vi "Get Types for Worker.vi"(11 "Worker VI In":refnum<vi>) -> (1 "Types":T2[](array[typedef]), 2 "Special Terminals":T1={"Action"=-1, "Init"=-1, "Tag"=-1, "State in"=-1, "State out"=-1, "Error"=-1}, 3 "Worker VI":refnum<vi>)   [LabVIEW 2020, in "FlexBlocks.lvlib"]
uses:
  FlexBlocks.lvlib
  Special Terminal Indices.ctl
  Worker Action.ctl
  <vilib>/Utility/Data Type/NI_Data Type.lvlib
  Terminal Direction.ctl
  Value Mode.ctl
  Special Terminal.ctl
  Type Descriptor.ctl
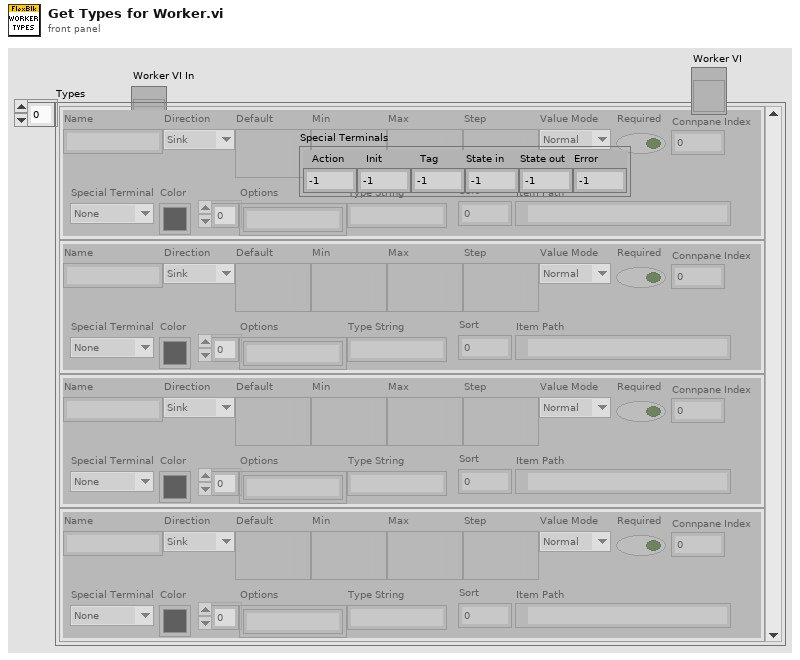
[diagram p1: front panel]
types:
  T1 = typedef "FlexBlocks.lvlib/Special Terminal Indices.ctl" = cluster{"Action":i32, "Init":i32, "Tag":i32, "State in":i32, "State out":i32, "Error":i32}
  T2 = typedef "FlexBlocks.lvlib/Type Descriptor.ctl" = cluster{"Name":string, "Direction":T3, "Default":variant, "Min":variant, "Max":variant, "Step":variant, "Value Mode":T4, "Required":bool, "Connpane Index":i32, "Special Terminal":T5, "Color":u32, "Options":string[], "Type String":string, "Sort":i32, "Item Path":path}
  T3 = typedef "FlexBlocks.lvlib/Terminal Direction.ctl" = enum16{"Sink", "Source"}
  T4 = typedef "FlexBlocks.lvlib/Value Mode.ctl" = enum16{"Normal", "Range", "Select"}
  T5 = typedef "FlexBlocks.lvlib/Special Terminal.ctl" = enum16{"None", "Action", "Init", "Tag", "State in", "State out", "Error"}
  T6 = typedef "FlexBlocks.lvlib/Worker Action.ctl" = enum16{"Start", "Work", "Stop"}
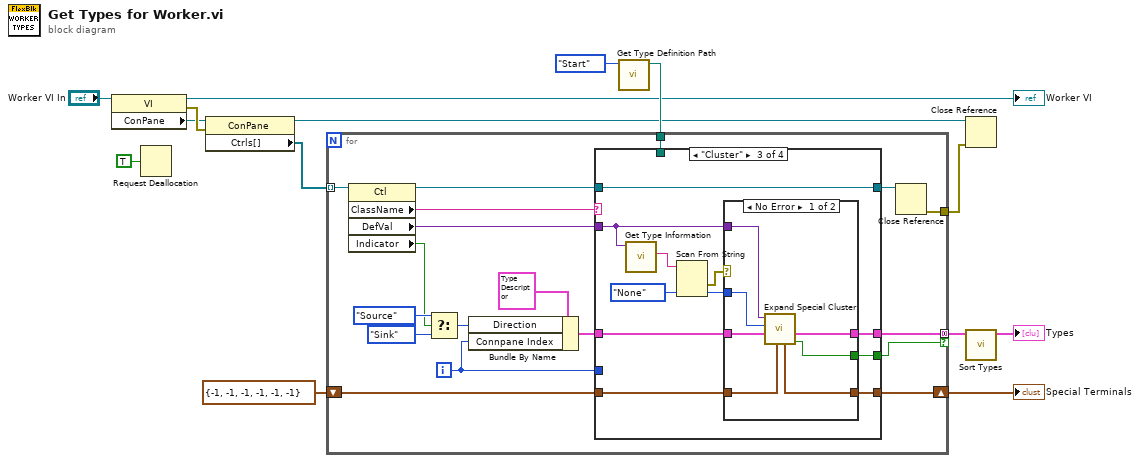
[diagram p0: block diagram]
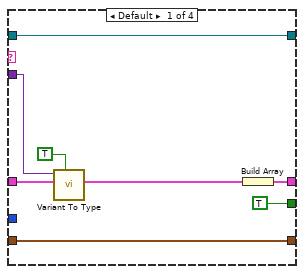
[diagram p2: hidden frame]
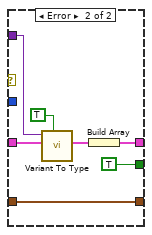
[diagram p4: hidden frame]
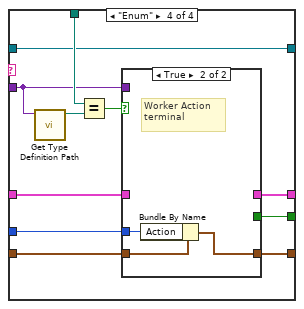
[diagram p5: hidden frame]
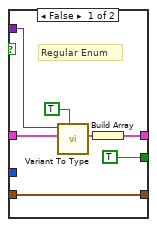
[diagram p6: hidden frame]
diagram:
  n1 = property class="VI"(reference="Worker VI In") -> (reference out=→"Worker VI":refnum<vi>, error out=w14:errorcluster, "ConPane"=w13:refnum<vi>)  [unwired: 1 in]
  n2 = Request Deallocation(TRUE ("flag")) -> ()
  n3 = property class="ConPane"(reference=w13, error in=w14) -> (reference out=w6:refnum<vi>, "Ctrls[]"=w10:refnum<vi>[])  [unwired: 1 out]
  n4 = call <vilib>:"Get Type Definition Path.vi"("variant"=Worker_Action."Start" ("Action")) -> ("type definition path"=w7:path)  [unwired: 9 in, 1 out]
  n5 = for {
    tunnel: w10 -> [w32] mode=indexing
    shift-right: [w18] -> w3
    shift-left: T1 {"Action"=-1, "Init"=-1, "Tag"=-1, "State in"=-1, "State out"=-1, "Error"=-1} ("Special Term Indices") -> [w19]
    tunnel: w7 -> [w17]
    tunnel: [w21] -> w4 mode=concatenating if=w20
    tunnel: [w15] -> w5
    i -> [w23]
    n6 = property class="Ctl"(reference=w32) -> (reference out=w30:refnum<vi>, "ClassName"=w31:string, "DefVal"=w29:variant, "Indicator"=w26:bool)  [unwired: 1 in, 1 out]
    n7 = Select(t=Terminal_Direction."Source" ("Direction"), s=w26, f=Terminal_Direction."Sink" ("Direction")) -> (s? t:f=w24:T3)
    n8 = Bundle By Name(cluster=T2 {"Name"="", "Direction"=enum."Sink", "Default"=variant, "Min"=variant, "Max"=variant, "Step"=variant, "Value Mode"=enum."Normal", "Required"=FALSE, "Connpane Index"=0, "Special Terminal"=enum."None", "Color"=0, "Options"=[], "Type String"="", "Sort"=0, "Item Path"=path ""} ("Type Descriptor"), "Direction"=w24, "Connpane Index"=w23) -> (w22:T2)
    n9 = case shown="\"Cluster\"" w31 {
      tunnel: w30 -> [w33 w41 w43 w68]
      tunnel: w29 -> [w39 _ w48 w71]
      tunnel: w23 -> [_ _ _ w73]
      tunnel: w22 -> [w40 _ w49 w74]
      tunnel: [w36 _ w47 w70] -> w21
      tunnel: [TRUE _ w46 w69] -> w20
      tunnel: w19 -> [w34 w42 w45 w76]
      tunnel: [w34 w42 w44 w72] -> w18
      tunnel: w17 -> [_ _ _ w77]
      tunnel: [w33 w41 w43 w68] -> w16
      frame Default {
        n10 = call "Variant To Type.vi"("Required? (F)"=TRUE, "Type In"=w40, "Value"=w39) -> ("Type"=w37:T2)  [unwired: 8 in]
        n11 = Build Array(w37) -> (w36:T2[])
      }
      frame "" {
      }
      frame "Cluster" {
        n12 = call <vilib>:"Get Type Information.vi"("variant"=w48) -> ("name"=w53:string)  [unwired: 6 in, 4 out]
        n13 = Scan From String(input string=w53, default 1=Special_Terminal."None" ("Special Terminal")) -> (error out=w51:errorcluster, output 1=w50:T5)  [unwired: 3 in, 2 out]
        n14 = case shown="No Error" w51 {
          tunnel: w50 -> [w54 _]
          tunnel: w49 -> [w60 w67]
          tunnel: w48 -> [w55 w66]
          tunnel: [w57 w63] -> w47
          tunnel: [w56 TRUE] -> w46
          tunnel: w45 -> [w59 w61]
          tunnel: [w58 w61] -> w44
          frame No Error {
            n15 = call "Expand Special Cluster.vi"("Special Term Indices In"=w59, "Starting TypeDesc"=w60, "Special Terminal"=w54, "Variant"=w55) -> ("Save Types?"=w56:bool, "Contained TypeDescs"=w57:T2[], "Special Term Indices"=w58:T1)  [unwired: 5 in]
          }
          frame Error {
            n16 = call "Variant To Type.vi"("Required? (F)"=TRUE, "Type In"=w67, "Value"=w66) -> ("Type"=w64:T2)  [unwired: 8 in]
            n17 = Build Array(w64) -> (w63:T2[])
          }
        }
      }
      frame "Enum" {
        n18 = call <vilib>:"Get Type Definition Path.vi"("variant"=w71) -> ("type definition path"=w78:path)  [unwired: 9 in, 1 out]
        n19 = Equal?(x=w77, y=w78) -> (x = y?=w75:bool)
        n20 = case shown="True" w75 {
          tunnel: w76 -> [w80 w88]
          tunnel: w74 -> [w85 _]
          tunnel: w73 -> [_ w87]
          tunnel: [w80 w86] -> w72
          tunnel: w71 -> [w84 _]
          tunnel: [w81 _] -> w70
          tunnel: [TRUE _] -> w69
          frame False {
            # "Regular Enum"
            n21 = call "Variant To Type.vi"("Required? (F)"=TRUE, "Type In"=w85, "Value"=w84) -> ("Type"=w82:T2)  [unwired: 8 in]
            n22 = Build Array(w82) -> (w81:T2[])
          }
          frame True {
            # "Worker Action terminal"
            n23 = Bundle By Name(cluster=w88, "Action"=w87) -> (w86:T1)
          }
        }
      }
    }
    n24 = Close Reference(reference=w16) -> (error out=w15:errorcluster)  [unwired: 1 in]
  }
  "Special Terminals" <- w3
  n25 = Close Reference(reference=w6, error in (no error)=w5) -> ()  [unwired: 1 out]
  n26 = call "Sort Types.vi"("Types"=w4) -> ("Sorted Types"=→"Types":T2[])  [unwired: 10 in]
